vi "Write Element of TestSteps.vi"(8 "error in (no error)":errorcluster, 9 "TestMeasureStep.lvclass":refnum<class "TestMeasureStep.lvclass">, 10 "index":i32, 11 "TestSeqClass in":refnum<class "TestSeqClass.lvclass">) -> (0 "error out":errorcluster, 3 "TestSeqClass out":refnum<class "TestSeqClass.lvclass">)   [LabVIEW 2019, in "TestSeqClass.lvclass"]
uses:
  TestSeqClass.lvclass
  TestMeasureStep/TestMeasureStep.lvclass
  TestSeqClass.lvclass/TestSeqClass.ctl
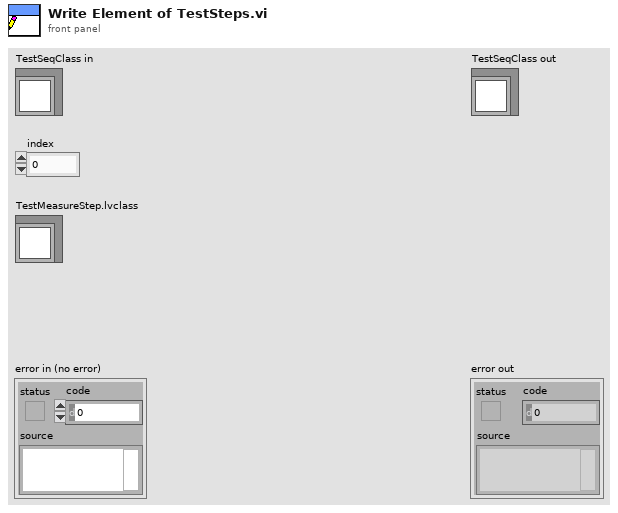
[diagram p1: front panel]
types:
  T1 = typedef "TestSeqType.ctl" = refnum<class "TestMeasureStep.lvclass">[]
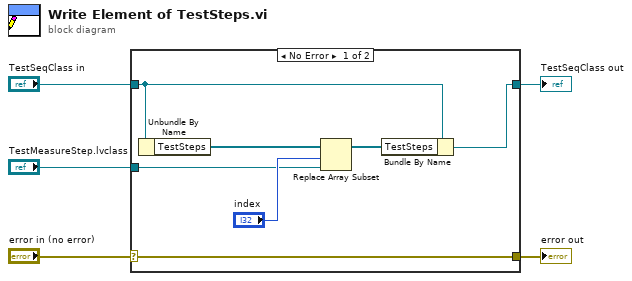
[diagram p0: block diagram]
diagram:
  n1 = case shown="No Error" "error in (no error)" {
    selector: "error in (no error)" -> [w12 w13]
    tunnel: [w12 w13] -> w4
    tunnel: [w11 w14] -> w2
    tunnel: "TestSeqClass in" -> [w10 w14]
    tunnel: "TestMeasureStep.lvclass" -> [w6 _]
    frame No Error {
      n2 = Unbundle By Name(w10) -> ("TestSteps"=w9:T1)
      n3 = Replace Array Subset(array=w9, new element=w6, index="index") -> (w8:T1)
      n4 = Bundle By Name(cluster=w10, "TestSteps"=w8) -> (w11:refnum<class "TestSeqClass.lvclass">)
    }
    frame Error {
    }
  }
  "error out" <- w4
  "TestSeqClass out" <- w2
